vi "enable.vi"(8 "error in (no error)":errorcluster, 11 "GenericEmissionSensor in":refnum<class "GenericDetector.lvclass">) -> (0 "error out":errorcluster, 3 "GenericEmissionSensor out":refnum<class "GenericDetector.lvclass">)   [LabVIEW 2010, in "GenericDetector.lvclass"]
uses:
  GenericDetector.lvclass
  status_enum.ctl
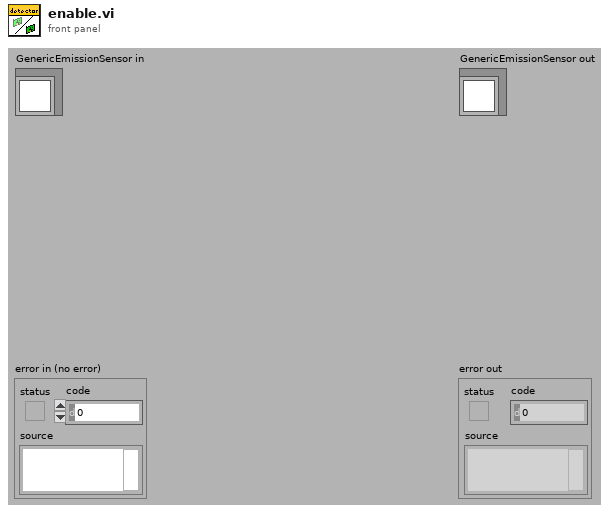
[diagram p1: front panel]
types:
  T1 = typedef "GenericDetector.lvclass/status_enum.ctl" = enum16{"disabled", "enabled"}
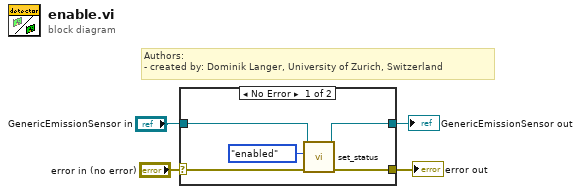
[diagram p0: block diagram]
diagram:
  # "Authors: \n- created by: Dominik Langer, University of Zurich, Switzerland"
  n1 = case shown="No Error" "error in (no error)" {
    selector: "error in (no error)" -> [w7 w11]
    tunnel: [w6 w11] -> w3
    tunnel: [w8 w10] -> w1
    tunnel: "GenericEmissionSensor in" -> [w9 w10]
    frame No Error {
      n2 = call-dynamic "set_status.vi"("error in (no error)"=w7, "status"=status_enum."enabled", "GenericEmissionSensor.lvclass in"=w9) -> ("error out"=w6:errorcluster, "GenericEmissionSensor.lvclass out"=w8:refnum<class "GenericDetector.lvclass">)  [unwired: 7 out]
    }
    frame Error {
    }
  }
  "error out" <- w3
  "GenericEmissionSensor out" <- w1
